vi "matrix_final (SubVI).vi"(10 "element 2":dbl[](array[numeric]), 11 "element":dbl[](array[numeric])) -> (3 "Real Matrix":T1)   [LabVIEW 2014]
uses:
  <vilib>/Analysis/Matrix/Datatypes/RealMatrix.ctl
  <vilib>/Analysis/Matrix/NI_Matrix.lvlib
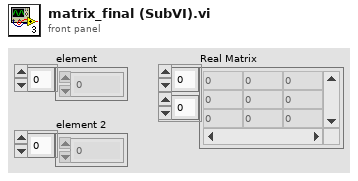
[diagram p1: front panel]
types:
  T1 = typedef "NI_Matrix.lvlib/RealMatrix.ctl" = dbl[][]
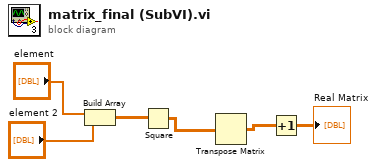
[diagram p0: block diagram]
diagram:
  n1 = Build Array("element", "element 2") -> (w1:T1)
  n2 = Square(x=w1) -> (x^2=w2:T1)
  n3 = Transpose Matrix(1:w2) -> (0:w3:T1)
  n4 = Increment(x=w3) -> (x+1=→"Real Matrix":T1)
